vi "Commit Prompt.vi"(9 "Path Statuses":T1[](array[typedef]), 10 "Branches":string[](array[string]), 11 "Branch":string) -> (0 "Commit Message":string, 1 "Paths":string[](array[string]), 2 "New Branch":string, 3 "Cancelled":bool)   [LabVIEW 2020, in "VolatusGUI.lvlib" / "Git Updater Module.lvclass"]
uses:
  Git Updater Module.lvclass
  Path Status.ctl
  Status.ctl
  lv-tree-tools/Tree Map/Tree Map/Extra Entry Info.ctl
  Git Updater Module.lvclass/Git Updater Module.ctl
  lv-tree-tools/Tree Map/Tree Map/Tree Map.lvclass
panel:
  out "Has Selected":bool
  out "Refresh":bool
  in  "New Branch Name":string
  out "Current Branch":string
  in  "Cancel":bool
  in  "Commit":bool
  in  "Create New Branch":bool
  in  "Select Versioned":bool
  in  "Select Unversioned":bool
  in  "Tree":string[](tree)
  in  "Select None":bool
  in  "Select All":bool
  in  "Message":string
  # "Commit to:"
  # "Select:"
  # "Commiting just tracks the changes locally, you need to do a push to send your local commits to the Git server."
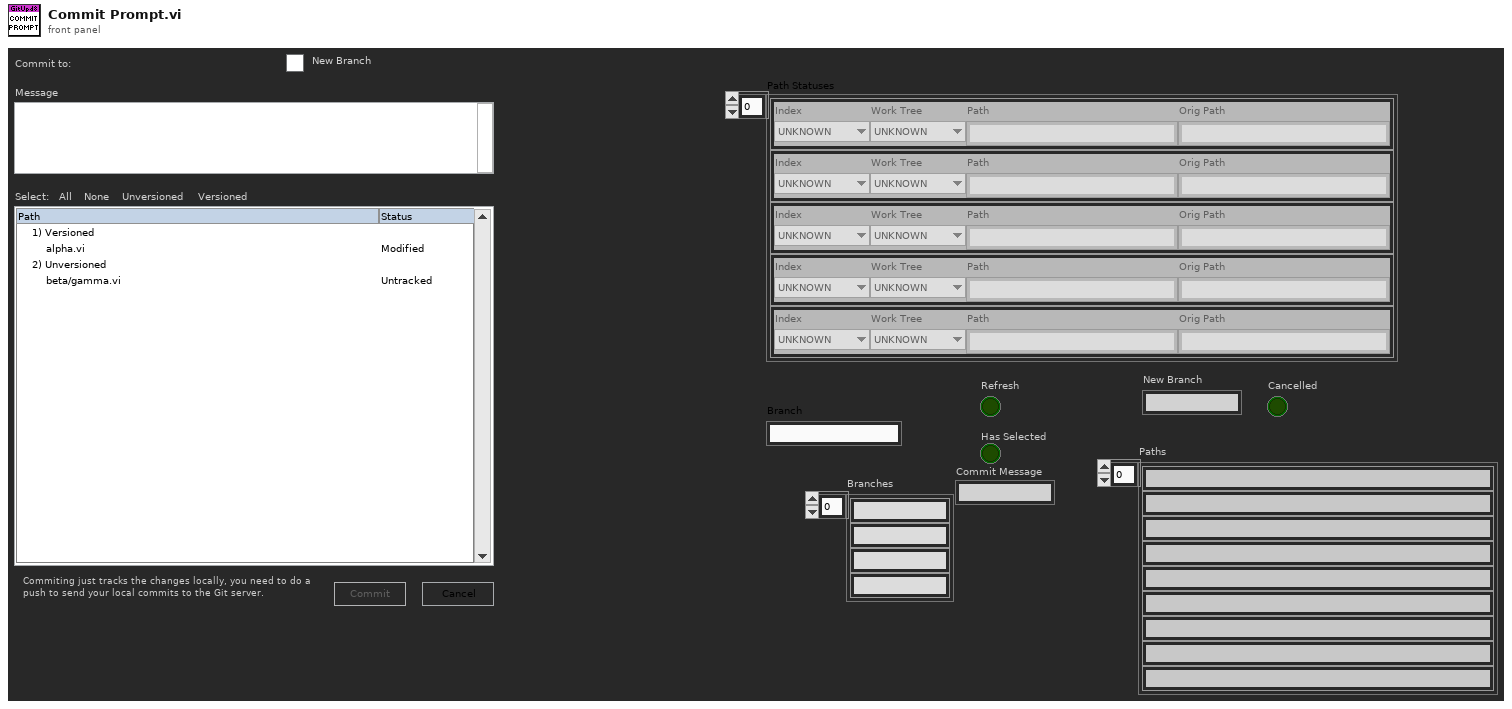
[diagram p1: front panel]
types:
  T1 = typedef "VolatusGUI.lvlib/Git Updater Module.lvclass/Path Status.ctl" = cluster{"Index":T2, "Work Tree":T2, "Path":string, "Orig Path":string}
  T2 = typedef "VolatusGUI.lvlib/Git Updater Module.lvclass/Status.ctl" = enum16{"UNKNOWN", "Unmodified", "Modified", "Added", "Deleted", "Renamed", "Unmerged", "Untracked", "Ignored"}
  T3 = enum8{"Enabled", "Disabled", "Disabled and Grayed Out"}
  T4 = typedef "LVPoint32TypeDef.ctl" = cluster{"Horizontal":i32, "Vertical":i32}
  T5 = typedef "Tree Map.lvlib/Tree Map.lvclass/Extra Entry Info.ctl" = cluster{"BG Color":u32, "Symbol":i32}
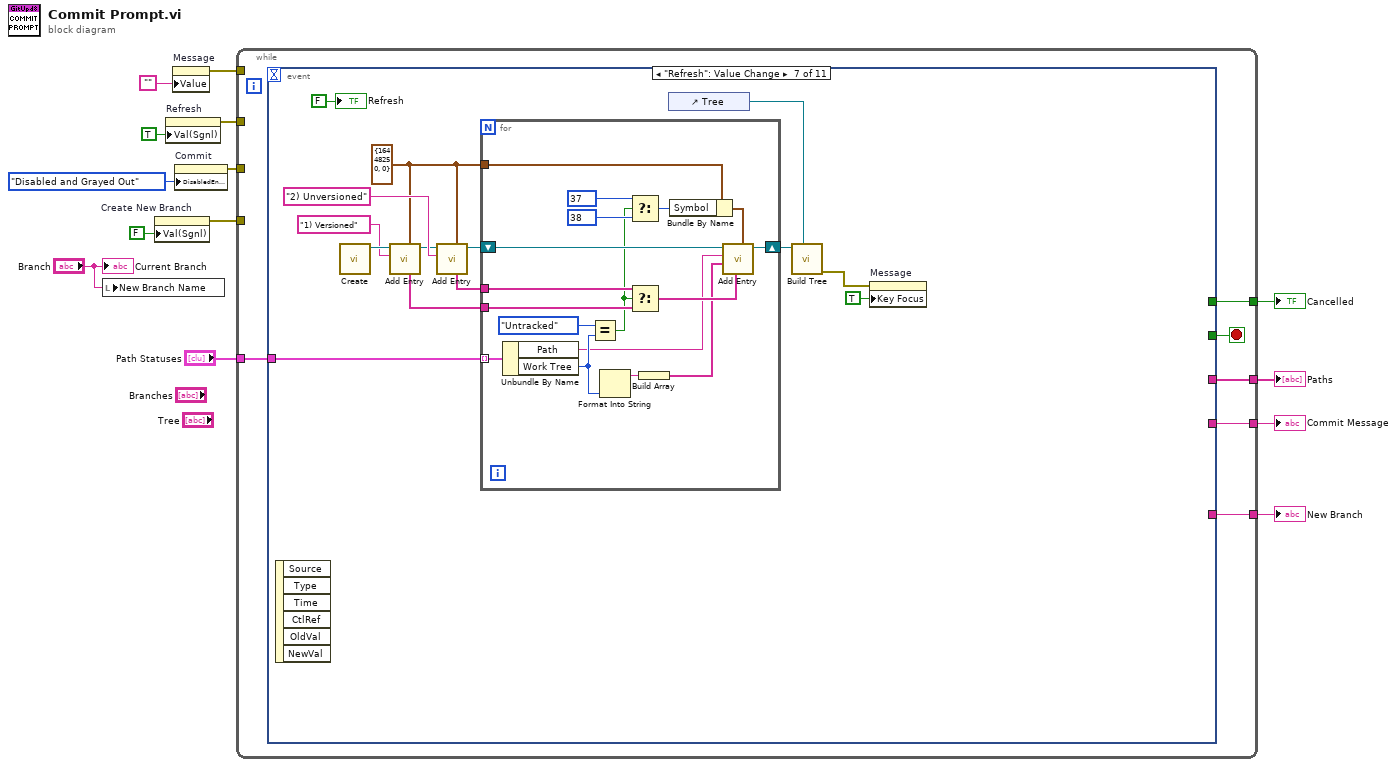
[diagram p0: block diagram]
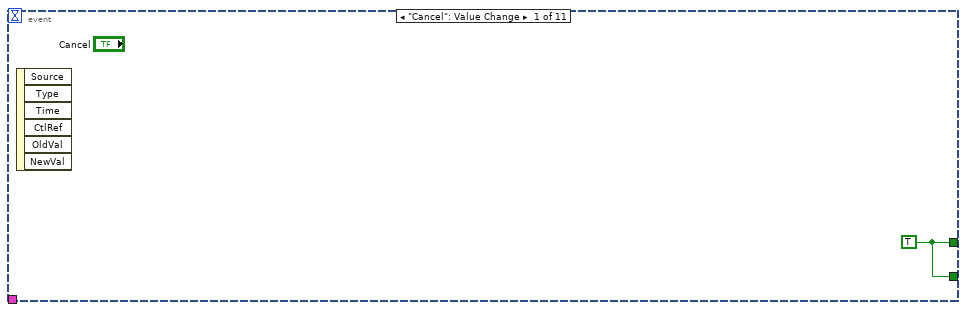
[diagram p2: hidden frame]
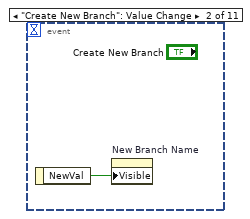
[diagram p3: hidden frame]
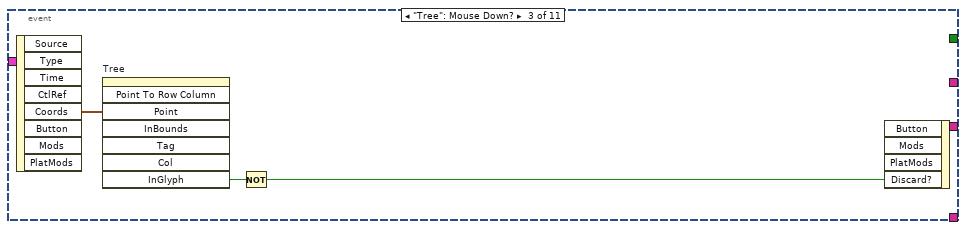
[diagram p4: hidden frame]
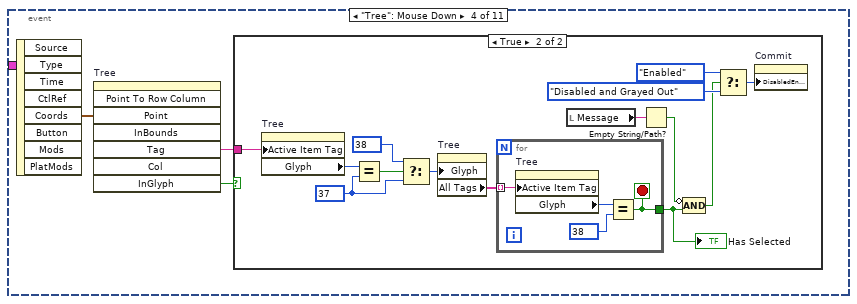
[diagram p5: hidden frame]
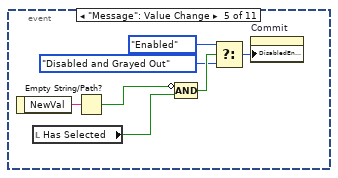
[diagram p7: hidden frame]
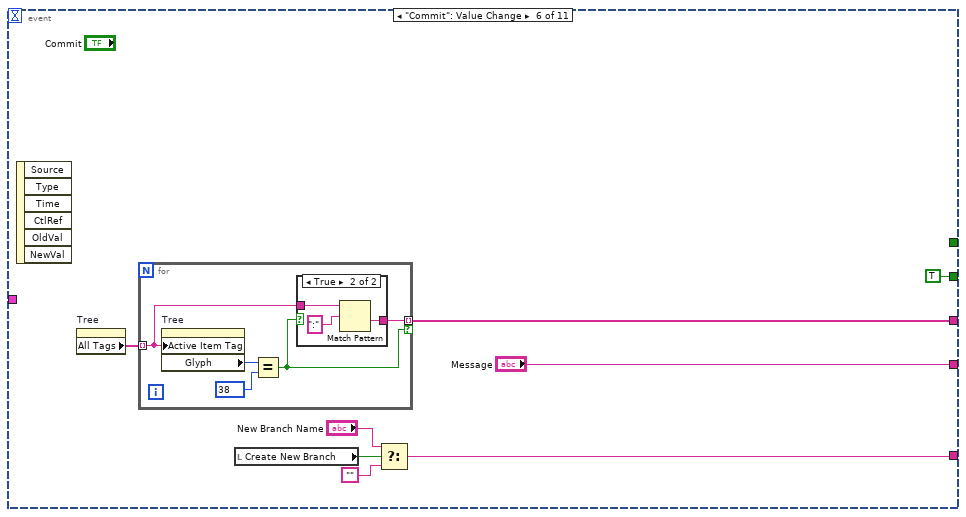
[diagram p8: hidden frame]
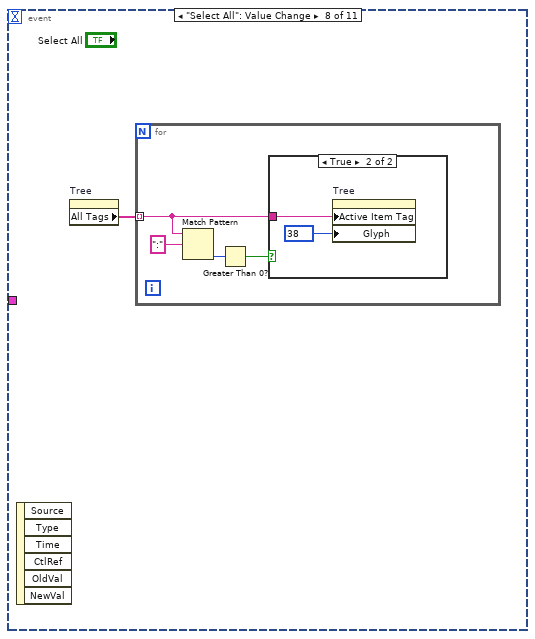
[diagram p10: hidden frame]
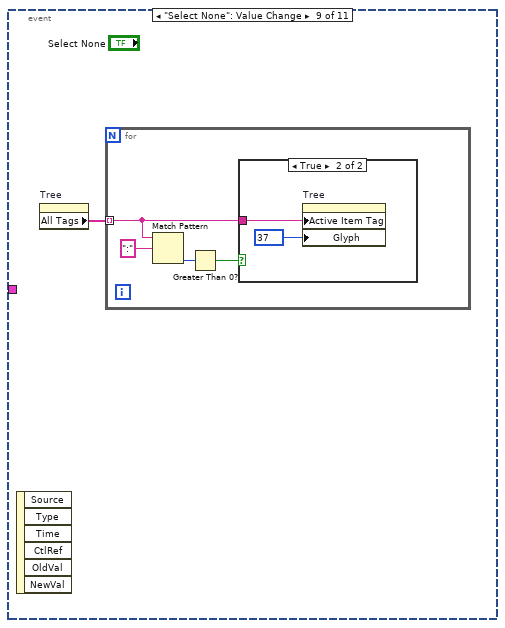
[diagram p12: hidden frame]
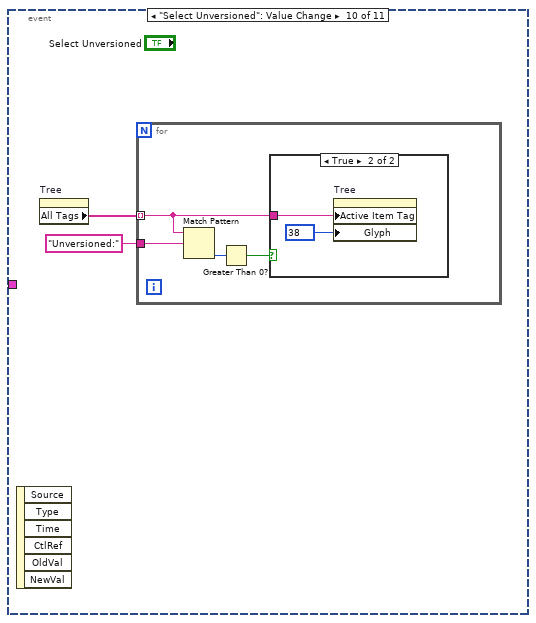
[diagram p14: hidden frame]
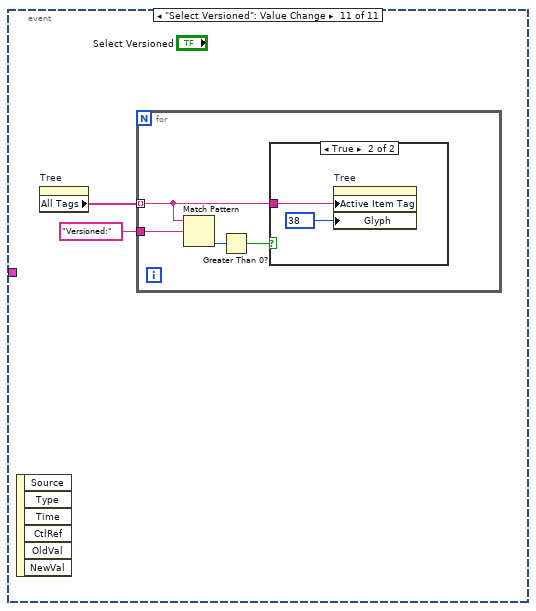
[diagram p16: hidden frame]
diagram:
  n1 = local write "New Branch Name"("Branch") -> ()
  n2 = property on="Create New Branch" class="Bool (strict)"("Val(Sgnl)"=FALSE ("Value (Signaling)")) -> (error out=w12:errorcluster)  [unwired: 2 in, 1 out]
  n3 = property on="Refresh" class="Bool (strict)"("Val(Sgnl)"=TRUE ("Value (Signaling)")) -> (error out=w9:errorcluster)  [unwired: 2 in, 1 out]
  n4 = property on="Message" class="Str"("Value"="") -> (error out=w5:errorcluster)  [unwired: 2 in, 1 out]
  n5 = property on="Commit" class="Bool"("DisabledEnum"=T3."Disabled and Grayed Out" ("Disabled")) -> (error out=w6:errorcluster)  [unwired: 2 in, 1 out]
  n6 = while {
    tunnel: [w20] -> w14
    tunnel: w12 -> [_]
    tunnel: w9 -> [_]
    tunnel: "Path Statuses" -> [w18]
    tunnel: w6 -> [_]
    tunnel: w5 -> [_]
    tunnel: [w17] -> w3
    tunnel: [w16] -> w2
    tunnel: [w15] -> w1
    stop <- w19 stop-if-true
    n7 = event shown="[6] \"Refresh\": Value Change" {
      selector: _ -> [_ _ _ _ _ _ _ _ _ _ _]
      dyn-events: _ -> [_ _ _ _ _ _ _ _ _ _ _]
      timeout: _ -> [_ _ _ _ _ _ _ _ _ _ _]
      tunnel: [w21 _ _ _ _ _ _ _ _ _ _] -> w20
      tunnel: [w21 _ _ _ _ TRUE _ _ _ _ _] -> w19
      tunnel: w18 -> [_ _ _ _ _ _ w82 _ _ _ _]
      tunnel: [_ _ _ _ _ w59 _ _ _ _ _] -> w17
      tunnel: [_ _ _ _ _ w55 _ _ _ _ _] -> w16
      tunnel: [_ _ _ _ _ "Message" _ _ _ _ _] -> w15
      event "Cancel": Value Change {
        w21 = TRUE
        n8 = event-data() -> ()  [unwired: 1 in, 6 out]
      }
      event "Create New Branch": Value Change {
        n9 = event-data() -> ("NewVal"=w22:bool)  [unwired: 1 in]
        n10 = property on="New Branch Name" class="Str"("Visible"=w22) -> ()  [unwired: 2 in, 2 out]
      }
      event "Tree": Mouse Down? {
        n11 = event-data() -> ("Coords"=w25:T4)  [unwired: 1 in, 7 out]
        n12 = invoke on="Tree" class="Tree (strict)" method="Point To Row Column"("Point"=w25) -> ("InGlyph"=w24:bool)  [unwired: 7 in, 7 out]
        n13 = Not(x=w24) -> (.not. x?=w23:bool)
        n14 = event-data("Discard?"=w23) -> ()  [unwired: 4 in, 1 out]
      }
      event "Tree": Mouse Down {
        n15 = event-data() -> ("Coords"=w28:T4)  [unwired: 1 in, 7 out]
        n16 = invoke on="Tree" class="Tree (strict)" method="Point To Row Column"("Point"=w28) -> ("Tag"=w26:string, "InGlyph"=w27:bool)  [unwired: 7 in, 6 out]
        n17 = case shown="True" w27 {
          tunnel: w26 -> [_ w42]
          frame False {
          }
          frame True {
            w40 = 37
            n18 = property on="Tree" class="Tree (strict)"("Active Item Tag"=w42) -> ("Glyph"=w41:i32)  [unwired: 2 in, 2 out]
            n19 = Equal?(x=w41, y=w40) -> (x = y?=w39:bool)
            n20 = Select(t=38, s=w39, f=w40) -> (s? t:f=w37:i32)
            n21 = property on="Tree" class="Tree (strict)"("Glyph"=w37) -> ("All Tags"=w33:string[])  [unwired: 2 in, 2 out]
            n22 = for {
              tunnel: w33 -> [w46] mode=indexing
              tunnel: [w43] -> w35
              stop <- w43 stop-if-true
              n23 = property on="Tree" class="Tree (strict)"("Active Item Tag"=w46) -> ("Glyph"=w44:i32)  [unwired: 2 in, 2 out]
              n24 = Equal?(x=w44, y=38) -> (x = y?=w43:bool)
            }
            "Has Selected" <- w35
            n25 = local read "Message"() -> (w36:string)
            n26 = Empty String/Path?(string/path=w36) -> (empty?=w34:bool)
            n27 = Compound Arithmetic op=AND(invert w34, w35) -> (w30:bool)
            n28 = Select(t=T3."Enabled" ("Disabled"), s=w30, f=T3."Disabled and Grayed Out" ("Disabled")) -> (s? t:f=w29:T3)
            n29 = property on="Commit" class="Bool"("DisabledEnum"=w29) -> ()  [unwired: 2 in, 2 out]
          }
        }
      }
      event "Message": Value Change {
        n30 = event-data() -> ("NewVal"=w53:string)  [unwired: 1 in]
        n31 = local read "Has Selected"() -> (w47:bool)
        n32 = Empty String/Path?(string/path=w53) -> (empty?=w48:bool)
        n33 = Compound Arithmetic op=AND(invert w48, w47) -> (w52:bool)
        n34 = Select(t=T3."Enabled" ("Disabled"), s=w52, f=T3."Disabled and Grayed Out" ("Disabled")) -> (s? t:f=w51:T3)
        n35 = property on="Commit" class="Bool"("DisabledEnum"=w51) -> ()  [unwired: 2 in, 2 out]
      }
      event "Commit": Value Change {
        n36 = event-data() -> ()  [unwired: 1 in, 6 out]
        n37 = property on="Tree" class="Tree (strict)"() -> ("All Tags"=w61:string[])  [unwired: 2 in, 2 out]
        n38 = for {
          tunnel: w61 -> [w64] mode=indexing
          tunnel: [w63] -> w59 mode=indexing if=w62
          n39 = property on="Tree" class="Tree (strict)"("Active Item Tag"=w64) -> ("Glyph"=w66:i32)  [unwired: 2 in, 2 out]
          n40 = Equal?(x=w66, y=38) -> (x = y?=w62:bool)
          n41 = case shown="True" w62 {
            tunnel: w64 -> [_ w69]
            tunnel: [_ w67] -> w63
            frame False {
            }
            frame True {
              n42 = Match Pattern(string=w69, regular expression=":") -> (after substring=w67:string)  [unwired: 1 in, 3 out]
            }
          }
        }
        n43 = local read "Create New Branch"() -> (w58:bool)
        n44 = Select(t="New Branch Name", s=w58, f="") -> (s? t:f=w55:string)
      }
      event "Refresh": Value Change {
        w72 = T5 {"BG Color"=16448250, "Symbol"=0} ("Extra Info")
        n45 = event-data() -> ()  [unwired: 1 in, 6 out]
        n46 = call "Create.vi"() -> ("Tree Map out"=w81:refnum<class "Tree Map.lvclass">)  [unwired: 10 in, 1 out]
        n47 = call "Add Entry.vi"("Extra Info"=w72, "Name"="1) Versioned", "Tree Map in"=w81) -> ("Tree Map out"=w77:refnum<class "Tree Map.lvclass">, "Hierarchy"=w79:string[])  [unwired: 6 in, 1 out]
        n48 = call "Add Entry.vi"("Extra Info"=w72, "Name"="2) Unversioned", "Tree Map in"=w77) -> ("Tree Map out"=w75:refnum<class "Tree Map.lvclass">, "Hierarchy"=w76:string[])  [unwired: 6 in, 1 out]
        n49 = for {
          tunnel: w82 -> [w100] mode=indexing
          tunnel: w79 -> [w97]
          tunnel: w76 -> [w98]
          shift-right: [w90] -> w74
          shift-left: w75 -> [w93]
          tunnel: w72 -> [w86]
          n50 = Unbundle By Name(w100) -> ("Path"=w92:string, "Work Tree"=w96:T2)
          n51 = Equal?(x=Status."Untracked", y=w96) -> (x = y?=w87:bool)
          n52 = Format Into String(w96) -> (resulting string=w99:string)  [unwired: 3 in, 1 out]
          n53 = Select(t=37, s=w87, f=38) -> (s? t:f=w85:i32)
          n54 = Select(t=w98, s=w87, f=w97) -> (s? t:f=w94:string[])
          n55 = Build Array(w99) -> (w91:string[])
          n56 = Bundle By Name(cluster=w86, "Symbol"=w85) -> (w84:T5)
          n57 = call "Add Entry.vi"("Extra Info"=w84, "Parent (None)"=w94, "Columns"=w91, "Name"=w92, "Tree Map in"=w93) -> ("Tree Map out"=w90:refnum<class "Tree Map.lvclass">)  [unwired: 4 in, 2 out]
        }
        n58 = control-ref of="Tree"() -> (w73:refnum<vi>)
        n59 = call "Build Tree.vi"("Tree"=w73, "Tree Map in"=w74) -> ("error out"=w71:errorcluster)  [unwired: 8 in, 1 out]
        n60 = property on="Message" class="Str"(error in=w71, "Key Focus"=TRUE) -> ()  [unwired: 1 in, 2 out]
        "Refresh" <- FALSE ("Refresh")
      }
      event "Select All": Value Change {
        n61 = event-data() -> ()  [unwired: 1 in, 6 out]
        n62 = property on="Tree" class="Tree (strict)"() -> ("All Tags"=w101:string[])  [unwired: 2 in, 2 out]
        n63 = for {
          tunnel: w101 -> [w105] mode=indexing
          n64 = Match Pattern(string=w105, regular expression=":") -> (offset past match=w103:i32)  [unwired: 1 in, 3 out]
          n65 = Greater Than 0?(x=w103) -> (x > 0?=w102:bool)
          n66 = case shown="True" w102 {
            tunnel: w105 -> [_ w106]
            frame False {
            }
            frame True {
              n67 = property on="Tree" class="Tree (strict)"("Active Item Tag"=w106, "Glyph"=38) -> ()  [unwired: 2 in, 2 out]
            }
          }
        }
      }
      event "Select None": Value Change {
        n68 = event-data() -> ()  [unwired: 1 in, 6 out]
        n69 = property on="Tree" class="Tree (strict)"() -> ("All Tags"=w108:string[])  [unwired: 2 in, 2 out]
        n70 = for {
          tunnel: w108 -> [w112] mode=indexing
          n71 = Match Pattern(string=w112, regular expression=":") -> (offset past match=w110:i32)  [unwired: 1 in, 3 out]
          n72 = Greater Than 0?(x=w110) -> (x > 0?=w109:bool)
          n73 = case shown="True" w109 {
            tunnel: w112 -> [_ w113]
            frame False {
            }
            frame True {
              n74 = property on="Tree" class="Tree (strict)"("Active Item Tag"=w113, "Glyph"=37) -> ()  [unwired: 2 in, 2 out]
            }
          }
        }
      }
      event "Select Unversioned": Value Change {
        n75 = event-data() -> ()  [unwired: 1 in, 6 out]
        n76 = property on="Tree" class="Tree (strict)"() -> ("All Tags"=w116:string[])  [unwired: 2 in, 2 out]
        n77 = for {
          tunnel: w116 -> [w120] mode=indexing
          tunnel: "Unversioned:" ("regular expression") -> [w117]
          n78 = Match Pattern(string=w120, regular expression=w117) -> (offset past match=w119:i32)  [unwired: 1 in, 3 out]
          n79 = Greater Than 0?(x=w119) -> (x > 0?=w118:bool)
          n80 = case shown="True" w118 {
            tunnel: w120 -> [_ w121]
            frame False {
            }
            frame True {
              n81 = property on="Tree" class="Tree (strict)"("Active Item Tag"=w121, "Glyph"=38) -> ()  [unwired: 2 in, 2 out]
            }
          }
        }
      }
      event "Select Versioned": Value Change {
        n82 = event-data() -> ()  [unwired: 1 in, 6 out]
        n83 = property on="Tree" class="Tree (strict)"() -> ("All Tags"=w124:string[])  [unwired: 2 in, 2 out]
        n84 = for {
          tunnel: w124 -> [w128] mode=indexing
          tunnel: "Versioned:" ("regular expression") -> [w125]
          n85 = Match Pattern(string=w128, regular expression=w125) -> (offset past match=w127:i32)  [unwired: 1 in, 3 out]
          n86 = Greater Than 0?(x=w127) -> (x > 0?=w126:bool)
          n87 = case shown="True" w126 {
            tunnel: w128 -> [_ w129]
            frame False {
            }
            frame True {
              n88 = property on="Tree" class="Tree (strict)"("Active Item Tag"=w129, "Glyph"=38) -> ()  [unwired: 2 in, 2 out]
            }
          }
        }
      }
    }
  }
  "Paths" <- w3
  "Cancelled" <- w14
  "New Branch" <- w2
  "Commit Message" <- w1
  "Current Branch" <- "Branch"
